vi "Test Record Failing Case Result.vi"(8 "error in (no error)":errorcluster, 11 "Result Model Result Recording Test in":refnum<class "Result Model Result Recording Test.lvclass">) -> (0 "error out":errorcluster, 3 "Result Model Result Recording Test out":refnum<class "Result Model Result Recording Test.lvclass">)   [LabVIEW 2020, in "Result Model Result Recording Test.lvclass"]
uses:
  Result Model Result Recording Test.lvclass
  source/Core/Result/Type.ctl
  source/Core/Result/Result.lvlib
  source/Core/Result/Status.ctl
  source/Core/Result/Result.ctl
  source/User Interface/Result Model/Result Model.lvclass
  ae2c71b8-32bb-49d1-8500-0119bfec74ff.vi
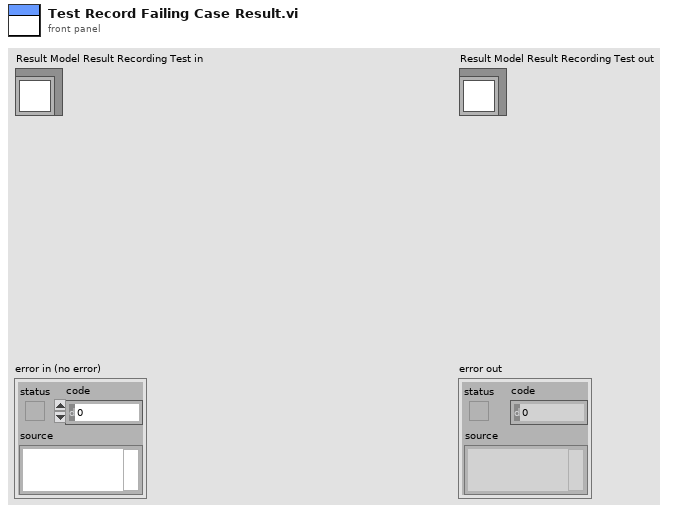
[diagram p1: front panel]
types:
  T1 = typedef "Result.lvlib/Result.ctl" = cluster{"Name":string, "Description":string, "Status":T2, "Result Type":T3, "Execution Time":dbl, "Data":cluster{"Expected":variant, "Actual":variant, "Delta":variant}}
  T2 = typedef "Result.lvlib/Status.ctl" = enum16{"", "Passed", "Failed", "Error", "Skipped", "Setup Error", "Broken", "Teardown Error"}
  T3 = typedef "Result.lvlib/Type.ctl" = enum16{"Test Case", "Test Suite", "Test Run", "Pass", "Fail", "Skip", "Pass if", "Fail if", "Pass if Error", "Fail if Error", "Pass if Equal", "Fail if Equal"}
  T4 = cluster{"Left Cell String":string, "Child Text":string[], "Child Tag":string, "Item Indent":i32, "Child Only?":bool, "Glyph Index":i32}[]
  T5 = cluster{"Left Cell String":string, "Child Text":string[], "Child Tag":string, "Item Indent":i32, "Child Only?":bool, "Glyph Index":i32}
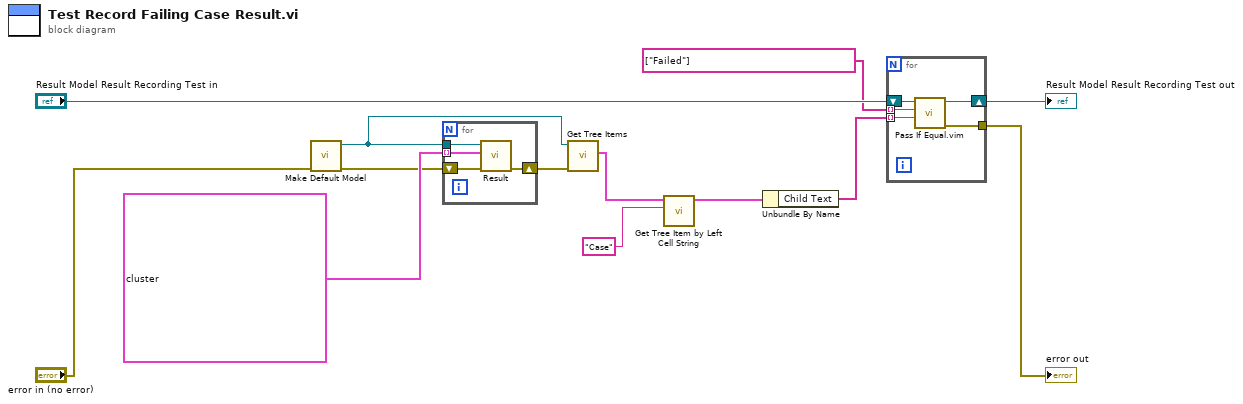
[diagram p0: block diagram]
diagram:
  n1 = call "Make Default Model.vi"("error in (no error)"="error in (no error)") -> ("error out"=w3:errorcluster, "Result Model out"=w1:refnum<class "Result Model.lvclass">)  [unwired: 9 in]
  n2 = for {
    tunnel: T1[] [{"Name"="Case.lvclass:Test Method.vi", "Description"="Failed:\nMessage", "Status"=enum."Failed", "Result Type"=enum."Test Case", "Execution Time"=0.107, "Data"={"Expected"=variant, "Actual"=variant, "Delta"=variant}}, {"Name"="Case.lvclass", "Description"="Failed:\nMessage", "Status"=enum."Failed", "Result Type"=enum."Test Suite", "Execution Time"=0.107, "Data"={"Expected"=variant, "Actual"=variant, "Delta"=variant}}] ("Array") -> [w17] mode=indexing
    tunnel: w1 -> [w14]
    shift-right: [w15] -> w2
    shift-left: w3 -> [w16]
    n3 = call-dynamic "Result.vi"("error in (no error)"=w16, "Results"=w17, "Result Model by Reference In"=w14) -> ("error out"=w15:errorcluster)  [unwired: 8 in]
  }
  n4 = call "Get Tree Items.vi"("error in (no error)"=w2, "Result Model by Reference In"=w1) -> ("Tree Items"=w13:T4)  [unwired: 8 in, 1 out]
  n5 = call "Get Tree Item by Left Cell String.vi"("Left Cell String"="Case", "Tree Items"=w13) -> ("Item"=w9:T5)  [unwired: 9 in]
  n6 = Unbundle By Name(w9) -> ("Child Text"=w8:string[])
  n7 = for {
    tunnel: w8 -> [w20] mode=indexing
    tunnel: [w19] -> w7
    tunnel: string[] ["Failed"] ("Child Text") -> [w18] mode=indexing
    shift-right: [w21] -> w10
    shift-left: "Result Model Result Recording Test in" -> [w22]
    n8 = call "Pass If Equal.vim"("Actual"=w20, "Expected"=w18, "LUnit Test Case In"=w22) -> ("error out"=w19:errorcluster, "LUnit Test Case Out"=w21:refnum<class "Result Model Result Recording Test.lvclass">)  [unwired: 7 in]
  }
  "error out" <- w7
  "Result Model Result Recording Test out" <- w10
